vi "programdata_write.vi"() -> (0 "error out":errorcluster)   [LabVIEW 2014]
uses:
  <vilib>/Utility/sysdir.llb/System Directory Type.ctl
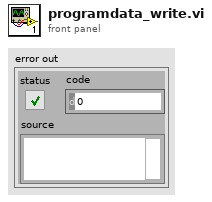
[diagram p1: front panel]
types:
  T1 = typedef "System Directory Type.ctl" = i32
  T2 = enum16{"open", "replace", "create", "open or create", "replace or create", "replace or create with confirmation"}
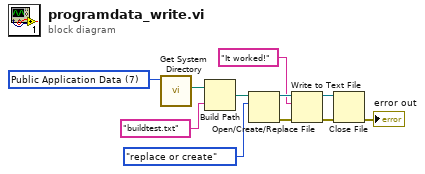
[diagram p0: block diagram]
diagram:
  w10 = T1 7 items=["User Home"=0, "User Desktop"=1, "User Documents"=2, "User Application Data"=3, "User Preferences"=4, "User Temporary"=5, "Public Documents"=6, "Public Application Data"=7, "Public Preferences"=8, "Public Cache"=13, "System Core Libraries"=9, "System Installed Libraries"=10, "Application Files"=11, "Boot Volume Root"=12] ("system directory type")
  n1 = call <vilib>:"Get System Directory.vi"("system directory type"=w10) -> ("system directory"=w9:path)  [unwired: 10 in]
  n2 = Build Path(base path=w9, name or relative path="buildtest.txt") -> (appended path=w7:path)
  n3 = Open/Create/Replace File(file path (use dialog)=w7, operation (0:open)=T2."replace or create") -> (refnum out=w6:refnum<file>, error out=w5:errorcluster)  [unwired: 4 in, 1 out]
  n4 = Write to Text File(file (use dialog)=w6, text="It worked!", error in=w5) -> (refnum out=w2:refnum<file>, error out=w3:errorcluster)  [unwired: 1 in, 1 out]
  n5 = Close File(refnum=w2, error in=w3) -> (error out=→"error out":errorcluster)  [unwired: 1 out]
